vi "Control value mapping.vi"(1 "Control In%":dbl, 2 "Demand Out%":dbl[](array[numeric]), 3 "Demand In%":dbl[](array[numeric])) -> (0 "Control Out%":dbl)   [LabVIEW 2017]
uses:
  <vilib>/Analysis/NI_AALPro.lvlib
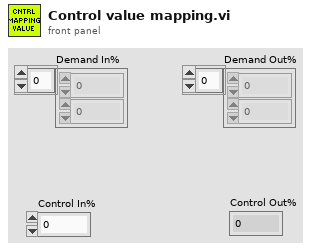
[diagram p1: front panel]
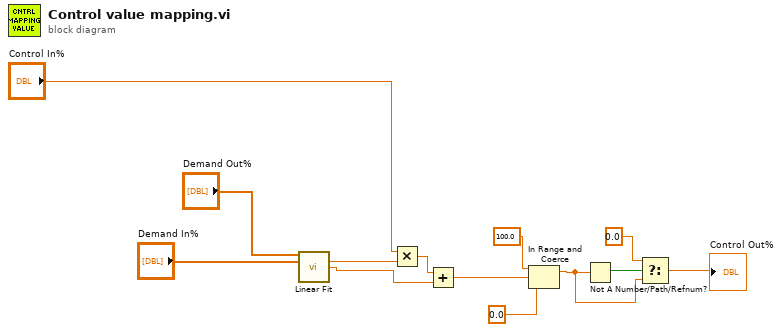
[diagram p0: block diagram]
diagram:
  n1 = call <vilib>:"Linear Fit.vi"("Y"="Demand Out%", "X"="Demand In%") -> ("slope"=w11:dbl, "intercept"=w8:dbl)  [unwired: 9 in, 3 out]
  n2 = Multiply(x="Control In%", y=w11) -> (x*y=w9:dbl)
  n3 = Add(x=w9, y=w8) -> (x+y=w7:dbl)
  n4 = In Range and Coerce(upper limit=100.0, x=w7, lower limit=0.0) -> (coerced(x)=w3:dbl)  [unwired: 1 out]
  n5 = Not A Number/Path/Refnum?(number/path/refnum=w3) -> (NaN/Path/Refnum?=w4:bool)
  n6 = Select(t=0.0, s=w4, f=w3) -> (s? t:f=→"Control Out%":dbl)
